vi "dataCleaning.vi"(0 "reference in":refnum<class "subject.lvclass">, 5 "error in (no error)":errorcluster) -> (14 "reference out":refnum<class "subject.lvclass">, 19 "error out":errorcluster)   [LabVIEW 2015, in "subject.lvclass"]
uses:
  subject.lvclass
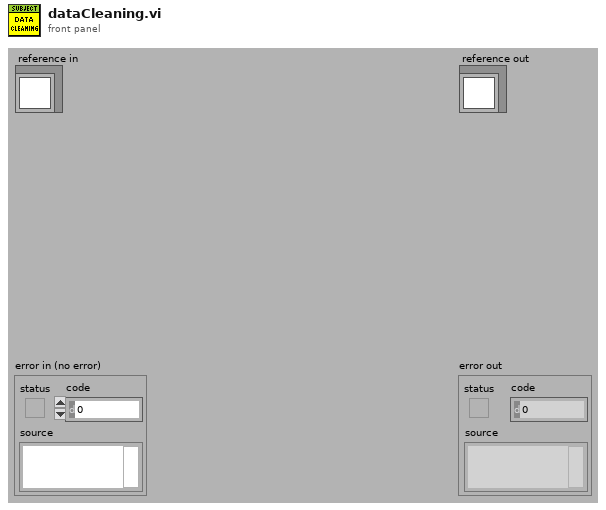
[diagram p1: front panel]
types:
  T1 = typedef "subject.lvclass/ObjectAttributesRef.ctl" = refnum<data-value>
  T2 = typedef "subject.lvclass/ObjectAttributes.ctl" = cluster{"MyAttribute":dbl, "data":cluster{"Ve_warm":dbl[], "time_warm":dbl[], "name":string, "phase":dbl[], "VCO2":dbl[], "VO2":dbl[], "PetCO2":dbl[], "RQ":dbl[], "HR":dbl[], "Ve_warm_inter":dbl[], "time_warm_inter":dbl[], "Ve_exer":dbl[], "time_exer":dbl[], "Ve_exer_inter":dbl[], "time_exer_inter":dbl[], "Ve":dbl[], "time":dbl[]}, "results_5l":cluster{"EOV":bool, "osci_amplitude":dbl[], "osci_width":dbl[], "peak_location":dbl[], "threshold":dbl, "width":i32}, "results_15percent":cluster{"EOV":bool, "osci_amplitude":dbl[], "osci_width":dbl[], "peak_location":dbl[], "threshold":dbl, "width":i32}, "supportData":cluster{"peaksAmplitude":dbl[], "iPeaksLocation":dbl[], "valesAmplitude":dbl[], "iValesLocation":dbl[], "threshold":dbl, "meanAmpl_warm":i32, "#_peaks":i32, "width":i32}, "results_user_selection":cluster{"EOV":bool, "osci_amplitude":dbl[], "osci_width":dbl[], "peak_location":dbl[], "threshold":dbl, "width":i32}}
  T3 = cluster{"Ve_warm":dbl[], "time_warm":dbl[], "name":string, "phase":dbl[], "VCO2":dbl[], "VO2":dbl[], "PetCO2":dbl[], "RQ":dbl[], "HR":dbl[], "Ve_warm_inter":dbl[], "time_warm_inter":dbl[], "Ve_exer":dbl[], "time_exer":dbl[], "Ve_exer_inter":dbl[], "time_exer_inter":dbl[], "Ve":dbl[], "time":dbl[]}
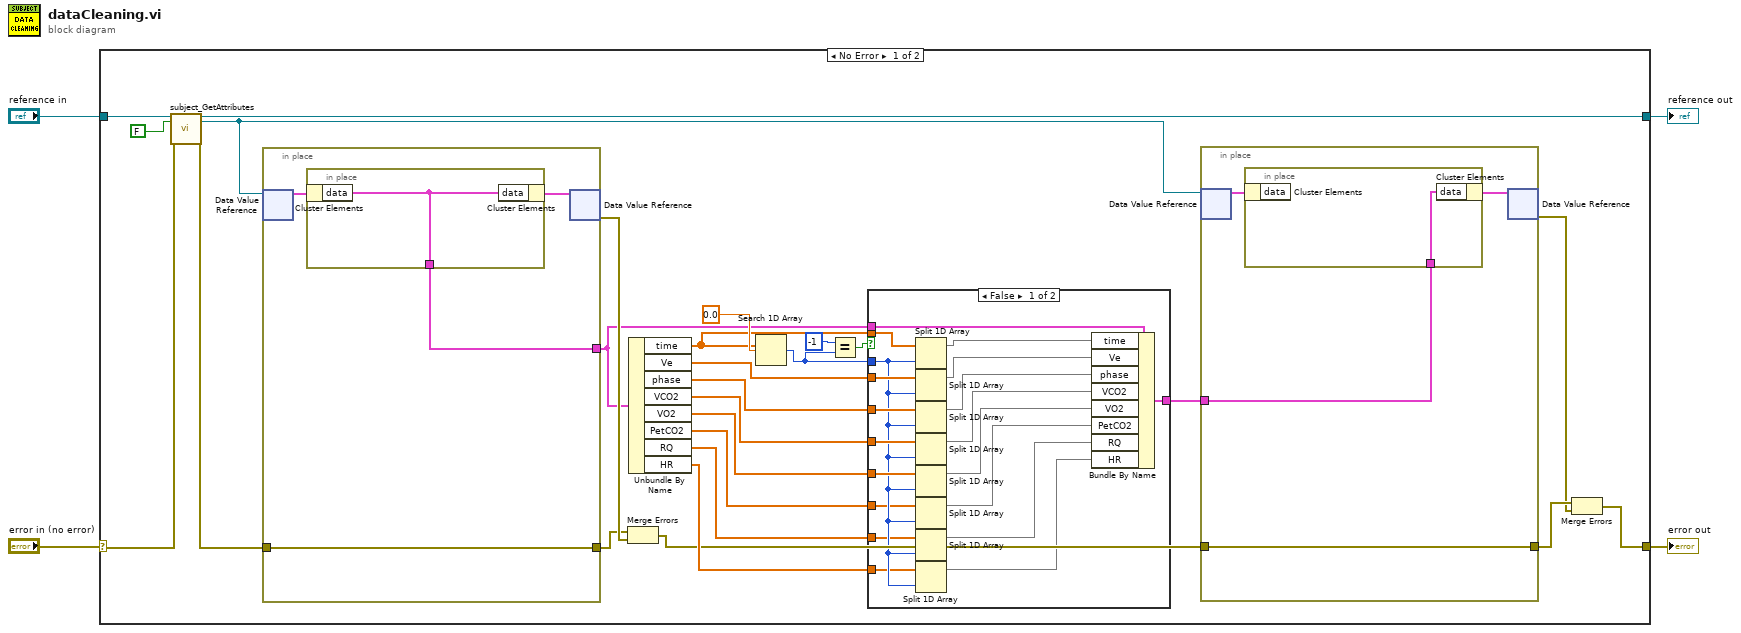
[diagram p0: block diagram]
diagram:
  n1 = case shown="No Error" "error in (no error)" {
    selector: "error in (no error)" -> [w26 w62]
    tunnel: [w9 w62] -> w3
    tunnel: [w24 w61] -> w1
    tunnel: "reference in" -> [w28 w61]
    frame No Error {
      n2 = call "subject_GetAttributes.vi"("reference in"=w28, "return data? (T)"=FALSE, "error in (no error)"=w26) -> ("reference out"=w24:refnum<class "subject.lvclass">, "attributes ref"=w8:T1, "error out"=w25:errorcluster)  [unwired: 13 in, 1 out]
      n3 = in-place {
        in-place-border: w25 -> [w57]
        in-place-border: [w57] -> w29
        in-place-border: [w56] -> w19
        n4 = in-place-dvr #1(w8) -> (w58:T2)  [unwired: 1 out]
        n5 = in-place {
          in-place-border: [w60] -> w56
          n6 = in-place-cluster #2(w58) -> ("data"=w60:T3)
          n7 = in-place-cluster #2("data"=w60) -> (w59:T2)
        }
        n8 = in-place-dvr #1(w59) -> (w30:errorcluster)  [unwired: 1 out]
      }
      n9 = Merge Errors(w29, w30) -> (w13:errorcluster)
      n10 = Unbundle By Name(w19) -> ("time"=w22:dbl[], "Ve"=w21:dbl[], "phase"=w20:dbl[], "VCO2"=w18:dbl[], "VO2"=w17:dbl[], "PetCO2"=w16:dbl[], "RQ"=w15:dbl[], "HR"=w14:dbl[])
      n11 = Search 1D Array(1D array=w22, element=0.0) -> (index of element=w6:i32)  [unwired: 1 in]
      n12 = Equal?(x=-1, y=w6) -> (x = y?=w7:bool)
      n13 = case shown="False" w7 {
        tunnel: w22 -> [w49 _]
        tunnel: w21 -> [w48 _]
        tunnel: w20 -> [w47 _]
        tunnel: w19 -> [w46 w50]
        tunnel: w18 -> [w42 _]
        tunnel: w17 -> [w41 _]
        tunnel: w6 -> [w40 _]
        tunnel: w16 -> [w39 _]
        tunnel: w15 -> [w38 _]
        tunnel: w14 -> [w37 _]
        tunnel: [w31 w50] -> w12
        frame False {
          n14 = Split 1D Array(array=w49, index=w40) -> (first subarray=w45:dbl[])  [unwired: 1 out]
          n15 = Split 1D Array(array=w48, index=w40) -> (first subarray=w44:dbl[])  [unwired: 1 out]
          n16 = Split 1D Array(array=w47, index=w40) -> (first subarray=w43:dbl[])  [unwired: 1 out]
          n17 = Split 1D Array(array=w42, index=w40) -> (first subarray=w36:dbl[])  [unwired: 1 out]
          n18 = Split 1D Array(array=w41, index=w40) -> (first subarray=w35:dbl[])  [unwired: 1 out]
          n19 = Split 1D Array(array=w39, index=w40) -> (first subarray=w34:dbl[])  [unwired: 1 out]
          n20 = Split 1D Array(array=w38, index=w40) -> (first subarray=w33:dbl[])  [unwired: 1 out]
          n21 = Split 1D Array(array=w37, index=w40) -> (first subarray=w32:dbl[])  [unwired: 1 out]
          n22 = Bundle By Name(cluster=w46, "time"=w45, "Ve"=w44, "phase"=w43, "VCO2"=w36, "VO2"=w35, "PetCO2"=w34, "RQ"=w33, "HR"=w32) -> (w31:T3)
        }
        frame True {
        }
      }
      n23 = in-place {
        in-place-border: w13 -> [w52]
        in-place-border: [w52] -> w11
        in-place-border: w12 -> [w51]
        n24 = in-place-dvr #3(w8) -> (w53:T2)  [unwired: 1 out]
        n25 = in-place {
          in-place-border: w51 -> [w55]
          n26 = in-place-cluster #4(w53) -> ()  [unwired: 1 out]
          n27 = in-place-cluster #4("data"=w55) -> (w54:T2)
        }
        n28 = in-place-dvr #3(w54) -> (w10:errorcluster)  [unwired: 1 out]
      }
      n29 = Merge Errors(w11, w10) -> (w9:errorcluster)
    }
    frame Error {
    }
  }
  "error out" <- w3
  "reference out" <- w1
